vi "Set for Channel FIFO Format.vi"(8 "error in (no error)":errorcluster, 11 "pcap_Parse_Build_CIF in":refnum<class "pcap_Parse_Build_CIF.lvclass">) -> (0 "error out":errorcluster, 3 "pcap_Parse_Build_CIF out":refnum<class "pcap_Parse_Build_CIF.lvclass">)   [LabVIEW 2021, in "pcap_Parse_Build_CIF.lvclass"]
doc: "If data is passed between elements where the global header is not present (such as using CIF channel FIFOs) the endian and the timestamp format must be set manually. The standard for these cases is little endian and ns format. This sets the defaults."
uses:
  pcap_Parse_Build_CIF.lvclass
  Typedef/File Format.ctl
  <vilib>/CIF Foundation/CIF Utilities/DataTypes/Typedef/Endian.ctl
  Typedef/Time Format.ctl
  pcap_Parse_Build_CIF.lvclass/pcap_Parse_Build_CIF.ctl
  <vilib>/CIF Foundation/CIF Utilities/DataTypes/DataTypes_CIF_U.lvlib
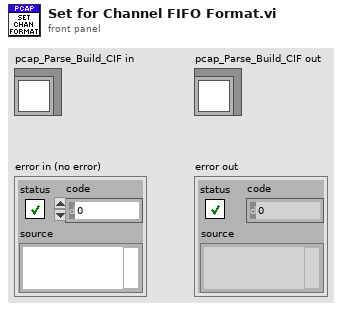
[diagram p1: front panel]
types:
  T1 = typedef "DataTypes_CIF_U.lvlib/Endian.ctl" = enum16{"Little Endian", "Big Endian"}
  T2 = typedef "pcap_Parse_Build_CIF.lvclass/File Format.ctl" = cluster{"Endian":T1, "Time Format":T3}
  T3 = typedef "pcap_Parse_Build_CIF.lvclass/Time Format.ctl" = enum16{"us", "ns"}
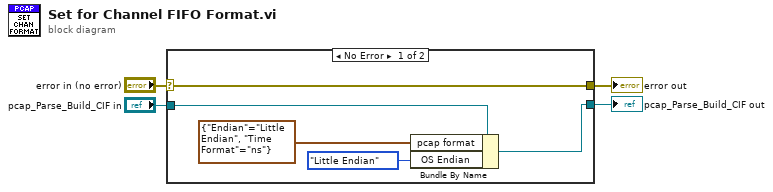
[diagram p0: block diagram]
diagram:
  n1 = case shown="No Error" "error in (no error)" {
    selector: "error in (no error)" -> [w9 w11]
    tunnel: [w9 w11] -> w3
    tunnel: [w7 w10] -> w1
    tunnel: "pcap_Parse_Build_CIF in" -> [w8 w10]
    frame No Error {
      n2 = Bundle By Name(cluster=w8, "pcap format"=T2 {"Endian"=enum."Little Endian", "Time Format"=enum."ns"}, "OS Endian"=Endian."Little Endian") -> (w7:refnum<class "pcap_Parse_Build_CIF.lvclass">)
    }
    frame Error {
    }
  }
  "error out" <- w3
  "pcap_Parse_Build_CIF out" <- w1
